vi "Send Command.vi"(6 "Line Break (T)?":bool=TRUE, 8 "error in (no error)":errorcluster, 9 "Delay (ms)":u32, 10 "Command":string, 11 "Controller States in":T1) -> (0 "error out":errorcluster, 3 "Controller States out":T1)   [LabVIEW 2019, in "Controller.lvlib"]
uses:
  Controller.lvlib
  Controller States.ctl
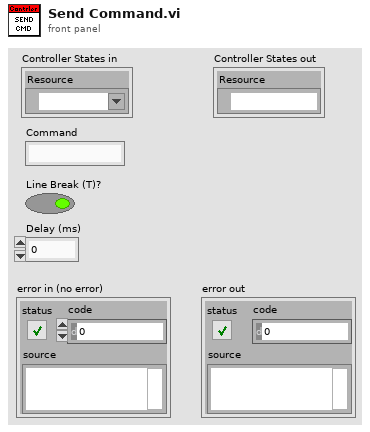
[diagram p1: front panel]
types:
  T1 = typedef "Controller.lvlib/Controller States.ctl" = cluster{"Resource":refnum<visa-resource-name>}
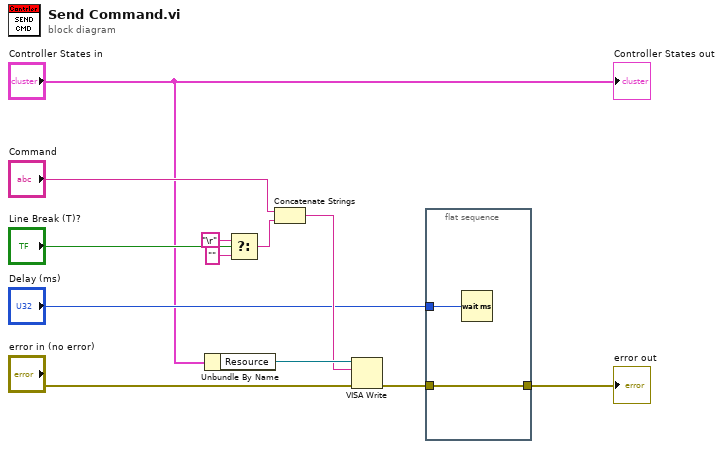
[diagram p0: block diagram]
diagram:
  n1 = Unbundle By Name("Controller States in") -> ("Resource"=w10:refnum<visa-resource-name>)
  n2 = Select(t="\r", s="Line Break (T)?", f="") -> (s? t:f=w5:string)
  n3 = Concatenate Strings("Command", w5) -> (w9:string)
  n4 = VISA Write(VISA resource name=w10, write buffer=w9, error in (no error)="error in (no error)") -> (error out=w8:errorcluster)  [unwired: 2 out]
  n5 = flat-sequence {
    tunnel: [w14] -> w1
    tunnel: w8 -> [w14]
    tunnel: "Delay (ms)" -> [w13]
    frame #0 {
      n6 = Wait (ms)(milliseconds to wait=w13) -> ()  [unwired: 1 out]
    }
  }
  "error out" <- w1
  "Controller States out" <- "Controller States in"
